vi "calib data profile string array to cluster array.vi"(11 "Data":string[][](array[string])) -> (1 "Array 2":T1[](array[typedef]), 2 "Array":T2[](array[typedef]), 3 "array w/ subset deleted":string[][](array[string]), 5 "Sr No.":i32[](array[numeric]))   [LabVIEW 2020]
uses:
  TypeDefs/Current Imaging Parameters.ctl
  TypeDefs/Current Calibration Parameters.ctl
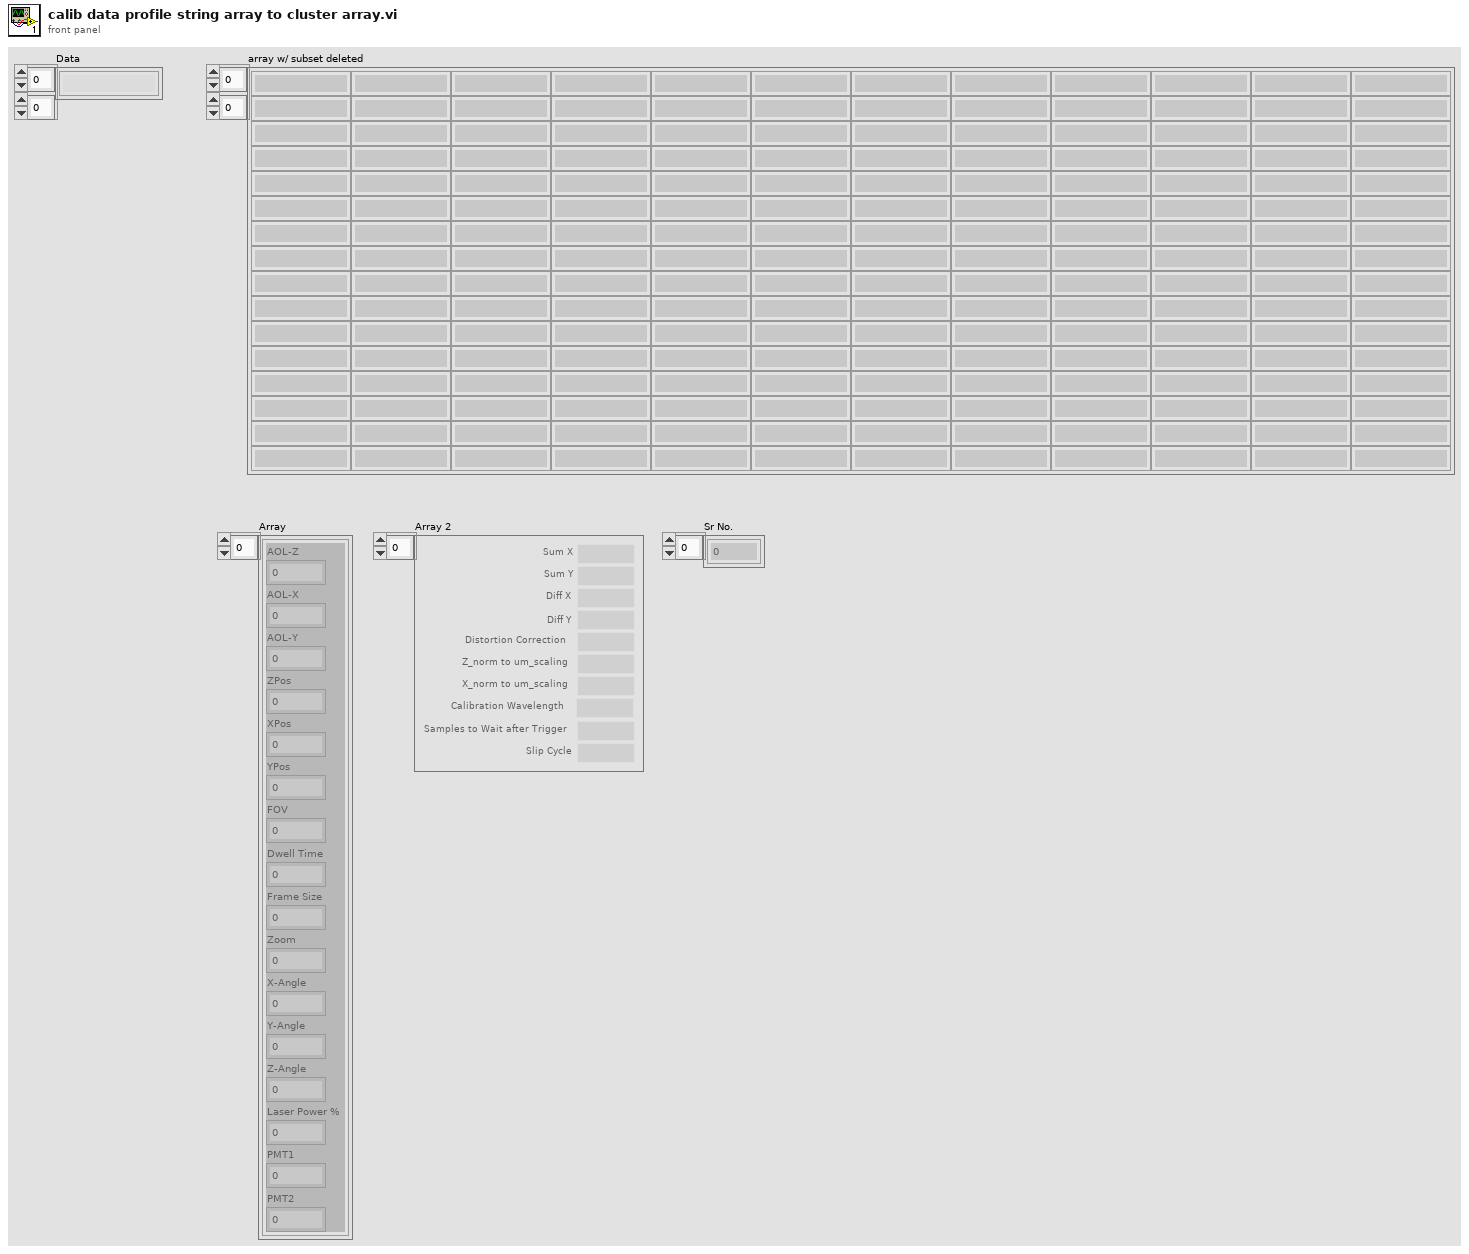
[diagram p1: front panel]
types:
  T1 = typedef "Current Calibration Parameters.ctl" = cluster{"Sum X":dbl, "Sum Y":dbl, "Diff X":dbl, "Diff Y":dbl, "Distortion Correction":dbl, "Z_norm to um_scaling":dbl, "X_norm to um_scaling":dbl, "Samples to Wait after Trigger":dbl, "Slip Cycle":dbl, "Calibration Wavelength":dbl}
  T2 = typedef "Current Imaging Parameters.ctl" = cluster{"AOL-Z":dbl, "AOL-X":dbl, "AOL-Y":dbl, "ZPos":dbl, "XPos":dbl, "YPos":dbl, "FOV":dbl, "Dwell Time":dbl, "Frame Size":dbl, "Zoom":dbl, "X-Angle":dbl, "Y-Angle":dbl, "Z-Angle":dbl, "Laser Power %":dbl, "PMT1":dbl, "PMT2":dbl}
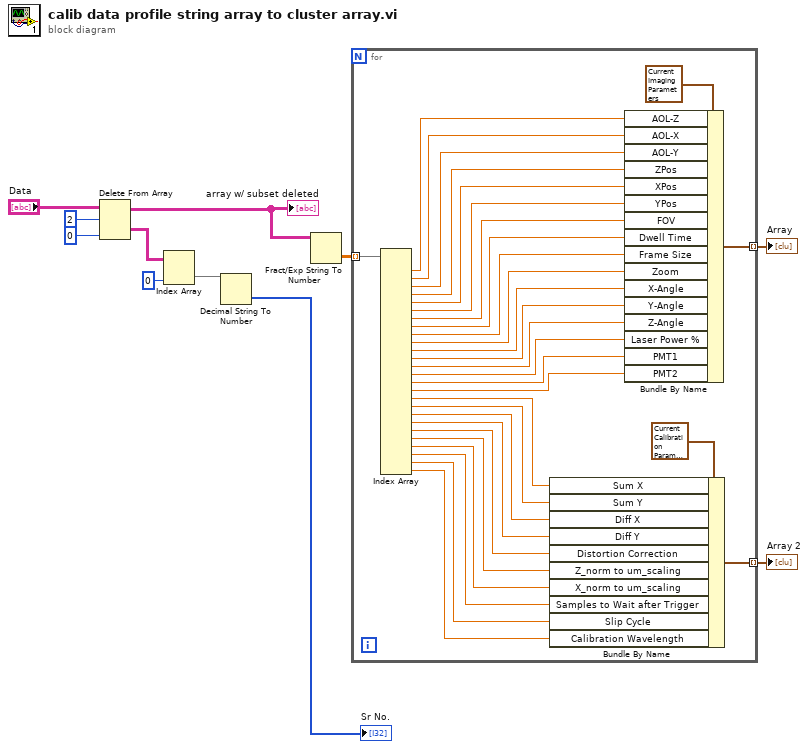
[diagram p0: block diagram]
diagram:
  n1 = Delete From Array(array="Data", length=2, index (col)=0 ("disabled index (col)")) -> (deleted portion=w4:string[][], array with subset deleted=w8:string[][])  [unwired: 1 in]
  "array w/ subset deleted" <- w8
  n2 = Index Array(array=w4, index (col)=0 ("disabled index (col)")) -> (element=w2:string[])  [unwired: 1 in]
  n3 = Decimal String To Number(string=w2) -> (number=→"Sr No.":i32[])  [unwired: 2 in, 1 out]
  n4 = Fract/Exp String To Number(string=w8) -> (number=w9:dbl[][])  [unwired: 3 in, 1 out]
  n5 = for {
    tunnel: w9 -> [w41] mode=indexing
    tunnel: [w13] -> w10 mode=indexing
    tunnel: [w12] -> w11 mode=indexing
    n6 = Index Array(array=w41) -> (element #1=w40:dbl, element #2=w39:dbl, element #3=w38:dbl, element #4=w37:dbl, element #5=w36:dbl, element #6=w35:dbl, element #7=w34:dbl, element #8=w33:dbl, element #9=w32:dbl, element #10=w31:dbl, element #11=w30:dbl, element #12=w29:dbl, element #13=w28:dbl, element #14=w27:dbl, element #15=w26:dbl, element #16=w25:dbl, element #17=w23:dbl, element #18=w22:dbl, element #19=w21:dbl, element #20=w20:dbl, element #21=w19:dbl, element #22=w18:dbl, element #23=w17:dbl, element #24=w16:dbl, element #25=w15:dbl, element #26=w14:dbl)  [unwired: 26 in]
    n7 = Bundle By Name(cluster=T1 {"Sum X"=0.0, "Sum Y"=0.0, "Diff X"=0.0, "Diff Y"=0.0, "Distortion Correction"=0.0, "Z_norm to um_scaling"=0.0, "X_norm to um_scaling"=0.0, "Samples to Wait after Trigger"=0.0, "Slip Cycle"=0.0, "Calibration Wavelength"=0.0} ("Calibration Parameters"), "Sum X"=w23, "Sum Y"=w22, "Diff X"=w21, "Diff Y"=w20, "Distortion Correction"=w19, "Z_norm to um_scaling"=w18, "X_norm to um_scaling"=w17, "Samples to Wait after Trigger"=w16, "Slip Cycle"=w15, "Calibration Wavelength"=w14) -> (w12:T1)
    n8 = Bundle By Name(cluster=T2 {"AOL-Z"=0.0, "AOL-X"=0.0, "AOL-Y"=0.0, "ZPos"=0.0, "XPos"=0.0, "YPos"=0.0, "FOV"=0.0, "Dwell Time"=0.0, "Frame Size"=0.0, "Zoom"=0.0, "X-Angle"=0.0, "Y-Angle"=0.0, "Z-Angle"=0.0, "Laser Power %"=0.0, "PMT1"=0.0, "PMT2"=0.0} ("Imaging Parameters"), "AOL-Z"=w40, "AOL-X"=w39, "AOL-Y"=w38, "ZPos"=w37, "XPos"=w36, "YPos"=w35, "FOV"=w34, "Dwell Time"=w33, "Frame Size"=w32, "Zoom"=w31, "X-Angle"=w30, "Y-Angle"=w29, "Z-Angle"=w28, "Laser Power %"=w27, "PMT1"=w26, "PMT2"=w25) -> (w13:T2)
  }
  "Array" <- w10
  "Array 2" <- w11
